vi "AlexeySRS865SweepAC.vi"(0 "VISA resource name":refnum<visa-resource-name>, 1 "Start Ampl":dbl caption="Start, V" format="%^.3e", 2 "Stop Ampl":dbl=1.0 caption="Stop, V" format="%^.5e", 3 "Step Ampl":dbl=0.001 caption="Step, V" format="%^.3e", 4 "Delay (s)":dbl=0.1 format="%.3f", 7 "Start Sweep":bool) -> (5 "Output Ampl":dbl)   [LabVIEW 2025]
doc: "Author: Scott Hannahs <sth@magnet.fsu.edu>\n\nThis software is licensed for use under the “MIT License\"\nCopyright (c) 2025 Scott Hannahs, sth@sth@magnet.sthnet.net\n\nPermission is hereby granted, free of charge, to any person obtaining a copy of this software and associated documentation files (the \"Software\"), to deal in the Software without restriction, including without limitation the rights to use, copy, modify, merge, publish, distribute, sublicense, and/or sell copies of the Software, and to permit persons to whom the Software is furnished to do so, subject to the following conditions: The above copyright notice and this permission notice shall be included in all copies or substantial portions of the Software.\n\nTHE SOFTWARE IS PROVIDED \"AS IS\", WITHOUT WARRANTY OF ANY KIND, EXPRESS OR IMPLIED, INCLUDING BUT NOT LIMITED TO THE WARRANTIES OF MERCHANTABILITY, FITNESS FOR A PARTICULAR PURPOSE AND NONINFRINGEMENT. IN NO EVENT SHALL THE AUTHORS OR COPYRIGHT HOLDERS BE LIABLE FOR ANY CLAIM, DAMAGES OR OTHER LIABILITY, WHETHER IN AN ACTION OF CONTRACT, TORT OR OTHERWISE, ARISING FROM, OUT OF OR IN CONNECTION WITH THE SOFTWARE OR THE USE OR OTHER DEALINGS IN THE SOFTWARE."
panel:
  in  "Pre-steps":dbl=5.0 format="%#_13g"
  in  "SetupBySoft":bool
  out "Calibration\nTime  (sec)":u32 format="%.1f"
  in  "Call Amp INIT":bool
  in  "Stop sweep":bool
  out "Initial Ampl":dbl
  in  "STOP VI":bool
  in  "Output Off":bool
  in  "Setup":bool
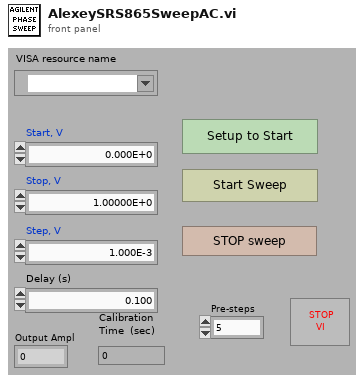
[diagram p1: front panel]
types:
  T1 = enum8{"Enabled", "Disabled", "Disabled and Grayed Out"}
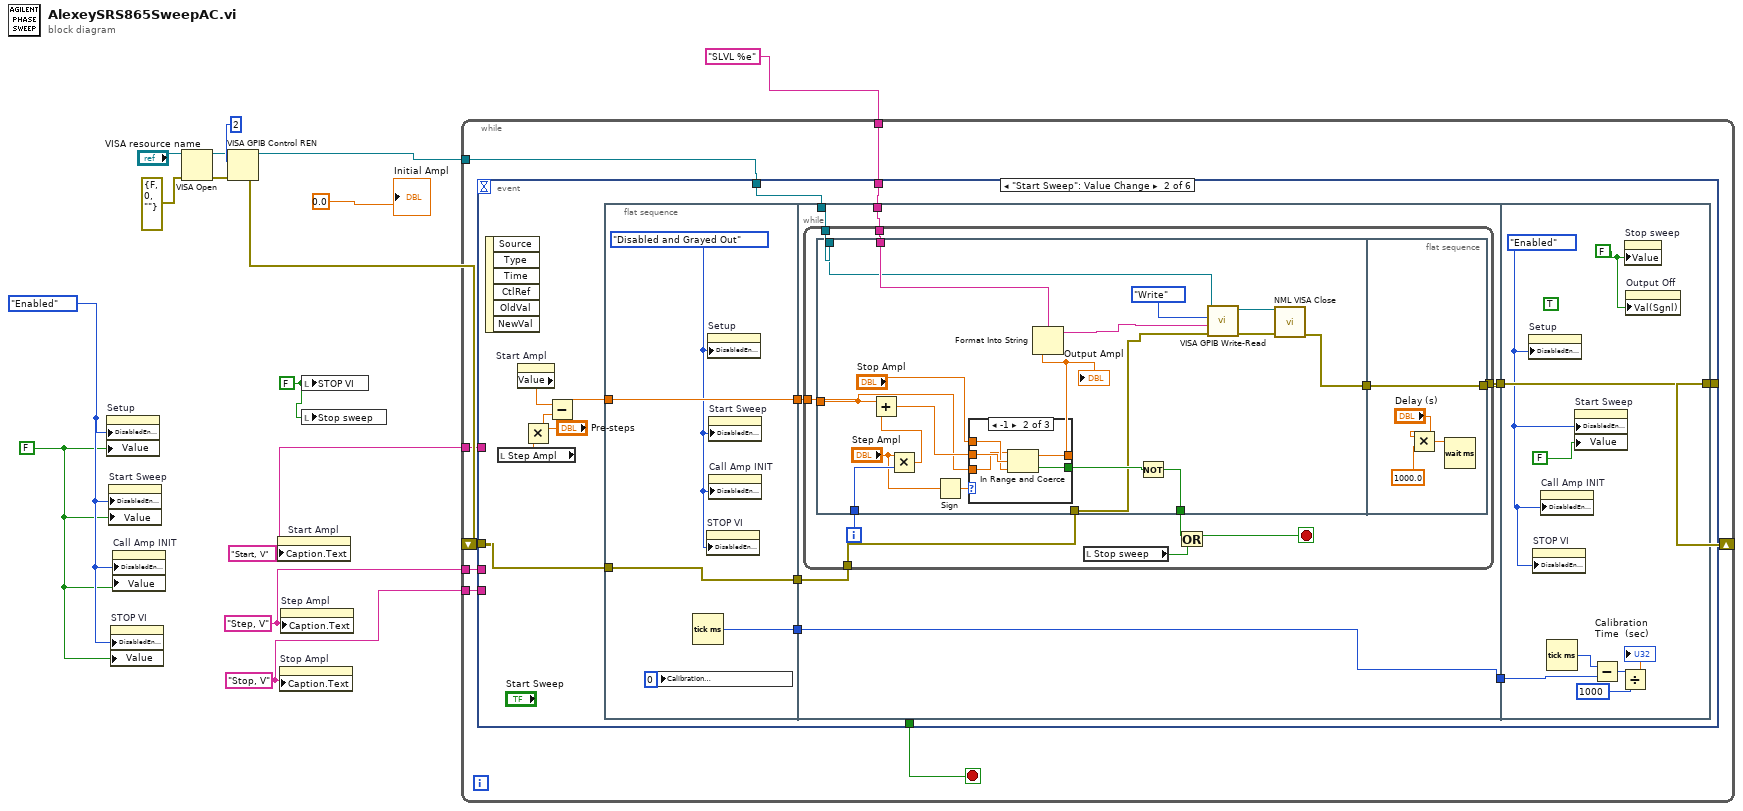
[diagram p0: block diagram]
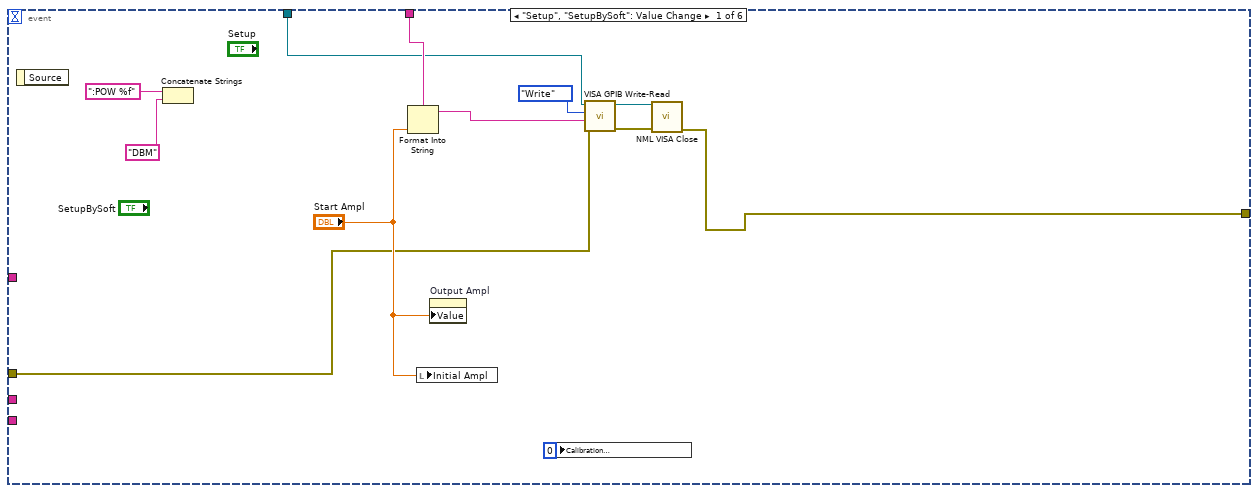
[diagram p2: hidden frame]
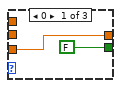
[diagram p3: hidden frame]
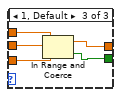
[diagram p4: hidden frame]
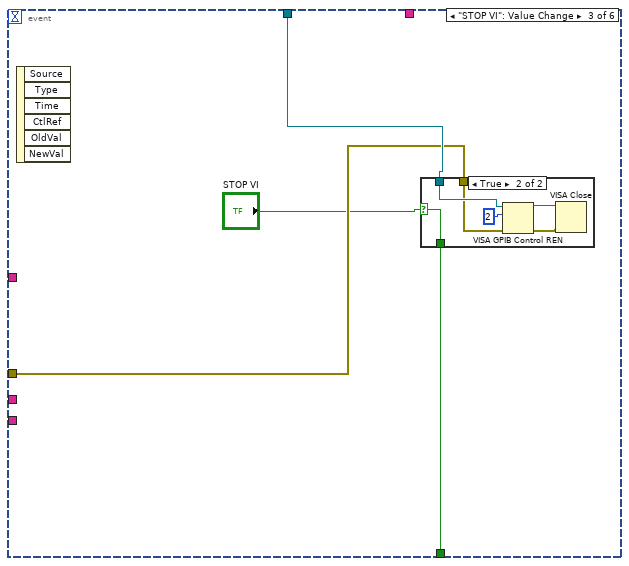
[diagram p5: hidden frame]
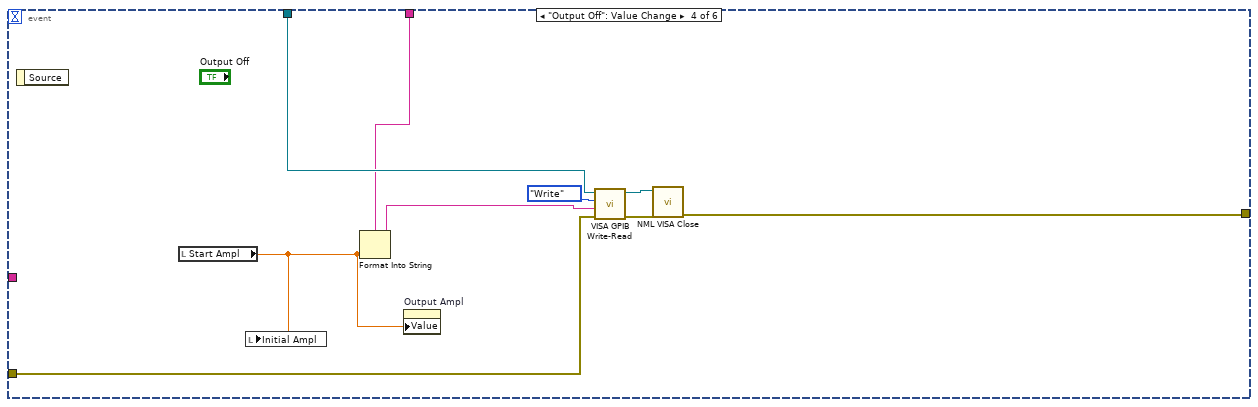
[diagram p7: hidden frame]
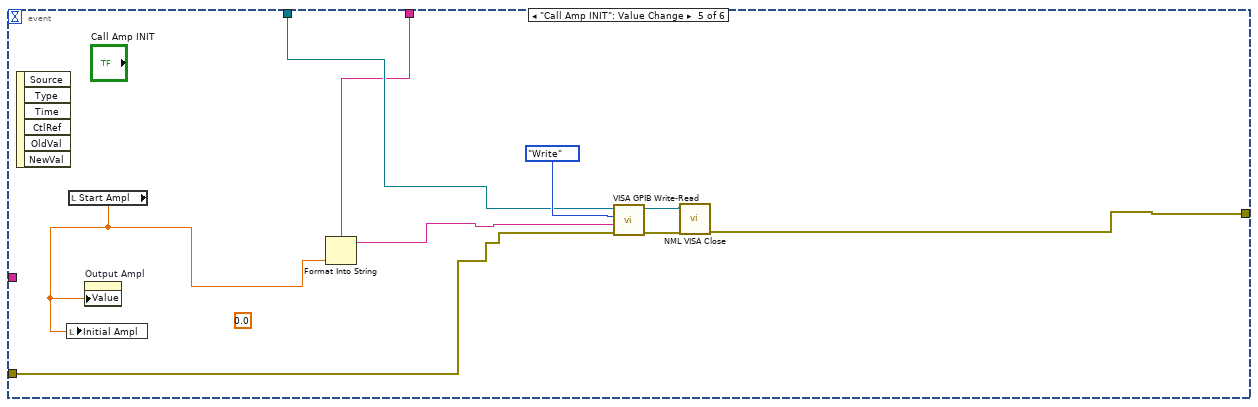
[diagram p8: hidden frame]
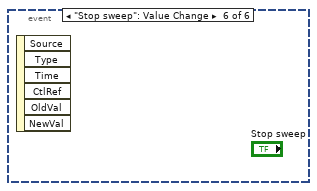
[diagram p9: hidden frame]
diagram:
  w4 = FALSE
  w5 = T1."Enabled" ("Disabled")
  w7 = "Stop, V" ("Label.Text")
  w8 = "Step, V" ("Label.Text")
  w9 = "Start, V" ("Label.Text")
  w6 = FALSE ("NewVal")
  n1 = property on="Setup" class="Bool"("DisabledEnum"=w5, "Value"=w4) -> ()  [unwired: 2 in, 2 out]
  n2 = property on="Start Sweep" class="Bool (strict)"("DisabledEnum"=w5, "Value"=w4) -> ()  [unwired: 2 in, 2 out]
  n3 = property on="STOP VI" class="Bool (strict)"("DisabledEnum"=w5, "Value"=w4) -> ()  [unwired: 2 in, 2 out]
  n4 = property on="Call Amp INIT" class="Bool"("DisabledEnum"=w5, "Value"=w4) -> ()  [unwired: 2 in, 2 out]
  n5 = VISA Open(error in (no error)=errorcluster {"status"=FALSE, "code"=0, "source"=""} ("error out"), VISA resource name="VISA resource name") -> (VISA resource name=w12:refnum<visa-resource-name>, error out=w13:errorcluster)  [unwired: 3 in]
  n6 = VISA GPIB Control REN(8:w13, 10:u16 2 ("mode"), 11:w12) -> (0:w10:errorcluster, 3:w3:refnum<visa-resource-name>)
  n7 = property on="Start Ampl" class="DigNum (strict)"("Caption.Text"=w9) -> ()  [unwired: 2 in, 2 out]
  n8 = property on="Stop Ampl" class="DigNum (strict)"("Caption.Text"=w7) -> ()  [unwired: 2 in, 2 out]
  n9 = property on="Step Ampl" class="DigNum (strict)"("Caption.Text"=w8) -> ()  [unwired: 2 in, 2 out]
  n10 = local write "STOP VI"(w6) -> ()
  n11 = local write "Stop sweep"(w6) -> ()
  n12 = while {
    shift-right: [w21] -> _
    shift-left: w10 -> [w23]
    tunnel: w3 -> [w22]
    tunnel: w9 -> [w19]
    tunnel: w8 -> [w18]
    tunnel: w7 -> [w17]
    tunnel: "SLVL %e" -> [w16]
    stop <- w20 stop-if-true
    n13 = event shown="[1] \"Start Sweep\": Value Change" {
      selector: _ -> [_ _ _ _ _ _]
      dyn-events: _ -> [_ _ _ _ _ _]
      timeout: _ -> [_ _ _ _ _ _]
      tunnel: w22 -> [w27 w49 w117 w133 w139 _]
      tunnel: [w24 w47 _ w125 w134 _] -> w21
      tunnel: w23 -> [w26 w48 w116 w130 w141 _]
      tunnel: [_ _ w114 _ _ _] -> w20
      tunnel: w19 -> [_ _ _ _ _ _]
      tunnel: w18 -> [_ _ _ _ _ _]
      tunnel: w17 -> [_ _ _ _ _ _]
      tunnel: w16 -> [w31 w38 _ w129 w137 _]
      event "Setup", "SetupBySoft": Value Change {
        n14 = event-data() -> ()  [unwired: 1 in, 1 out]
        n15 = Concatenate Strings(":POW %f", "DBM" ("string")) -> ()  [unwired: 1 out]
        n16 = Format Into String(format string=w31, "Start Ampl") -> (resulting string=w25:string)  [unwired: 2 in, 1 out]
        n17 = local write "Initial Ampl"("Start Ampl") -> ()
        n18 = property on="Output Ampl" class="DigNum (strict)"("Value"="Start Ampl") -> ()  [unwired: 2 in, 2 out]
        n19 = local write "Calibration\nTime  (sec)"(u32 0 ("Time Delay (ms)")) -> ()
        n20 = call "VISA GPIB Write-Read.vi"("error in (no error)"=w26, "Command"=w25, "Action"=enum16{"Write", "Read", "Write & Read"}."Write", "VISA resource name"=w27) -> ("error out"=w30:errorcluster, "dup VISA Session"=w29:refnum<visa-resource-name>)  [unwired: 4 in, 2 out]
        n21 = call "NML VISA Close.vi"("Error In"=w30, "VISA resource name"=w29) -> ("Error Out"=w24:errorcluster)  [unwired: 9 in]
      }
      event "Start Sweep": Value Change {
        n22 = event-data() -> ()  [unwired: 1 in, 6 out]
        n23 = local read "Step Ampl"() -> (w39:dbl)
        n24 = property on="Start Ampl" class="DigNum (strict)"() -> ("Value"=w40:dbl)  [unwired: 2 in, 2 out]
        n25 = Multiply(x="Pre-steps", y=w39) -> (x*y=w37:dbl)
        n26 = Subtract(x=w40, y=w37) -> (x-y=w41:dbl)
        n27 = flat-sequence {
          tunnel: w41 -> [w53]
          tunnel: w48 -> [w54]
          tunnel: [w54] -> w45
          tunnel: [w53] -> w44
          tunnel: [w51] -> w43
          tunnel: w49 -> [w60]
          tunnel: [w58] -> w46
          tunnel: w45 -> [w59]
          tunnel: w44 -> [w57]
          tunnel: w43 -> [w56]
          tunnel: [w56] -> w42
          tunnel: w38 -> [w55]
          tunnel: [w113] -> w47
          tunnel: w46 -> [w113]
          tunnel: w42 -> [w110]
          frame #0 {
            w52 = T1."Disabled and Grayed Out" ("Disabled")
            n28 = local write "Calibration\nTime  (sec)"(u32 0 ("Time Delay (ms)")) -> ()
            n29 = Tick Count (ms)() -> (millisecond timer value=w51:u32)
            n30 = property on="STOP VI" class="Bool (strict)"("DisabledEnum"=w52) -> ()  [unwired: 2 in, 2 out]
            n31 = property on="Setup" class="Bool"("DisabledEnum"=w52) -> ()  [unwired: 2 in, 2 out]
            n32 = property on="Start Sweep" class="Bool (strict)"("DisabledEnum"=w52) -> ()  [unwired: 2 in, 2 out]
            n33 = property on="Call Amp INIT" class="Bool"("DisabledEnum"=w52) -> ()  [unwired: 2 in, 2 out]
          }
          frame #1 {
            n34 = while {
              tunnel: w60 -> [w70]
              tunnel: w59 -> [w69]
              tunnel: [w68] -> w58
              tunnel: w57 -> [w67]
              tunnel: w55 -> [w61]
              i -> [w64]
              stop <- w63 stop-if-true
              n35 = flat-sequence {
                tunnel: w70 -> [w72]
                tunnel: w69 -> [w74]
                tunnel: w67 -> [w80]
                tunnel: [w88] -> w66
                tunnel: [w75] -> w65
                tunnel: w64 -> [w87]
                tunnel: w61 -> [w78]
                tunnel: [w104] -> w68
                tunnel: w65 -> [w104]
                frame #0 {
                  n36 = Multiply(x="Step Ampl", y=w87) -> (x*y=w86:dbl)
                  n37 = Add(x=w80, y=w86) -> (x+y=w82:dbl)
                  n38 = Sign(1:"Step Ampl") -> (0:w85:dbl)
                  n39 = case shown="-1" w85 {
                    tunnel: [FALSE w95 w96] -> w84
                    tunnel: [w90 w94 w97] -> w83
                    tunnel: w82 -> [_ w93 w100]
                    tunnel: "Stop Ampl" -> [_ w92 w99]
                    tunnel: w80 -> [w90 w91 w98]
                    frame 0 {
                    }
                    frame -1 {
                      n40 = In Range and Coerce(upper limit=w91, x=w93, lower limit=w92) -> (coerced(x)=w94:dbl, In Range?=w95:bool)
                    }
                    frame 1, Default {
                      n41 = In Range and Coerce(upper limit=w99, x=w100, lower limit=w98) -> (coerced(x)=w97:dbl, In Range?=w96:bool)
                    }
                  }
                  "Output Ampl" <- w83
                  n42 = Format Into String(format string=w78, w83) -> (resulting string=w73:string)  [unwired: 2 in, 1 out]
                  n43 = Not(x=w84) -> (.not. x?=w88:bool)
                  n44 = call "VISA GPIB Write-Read.vi"("error in (no error)"=w74, "Command"=w73, "Action"=enum16{"Write", "Read", "Write & Read"}."Write", "VISA resource name"=w72) -> ("error out"=w77:errorcluster, "dup VISA Session"=w76:refnum<visa-resource-name>)  [unwired: 4 in, 2 out]
                  n45 = call "NML VISA Close.vi"("Error In"=w77, "VISA resource name"=w76) -> ("Error Out"=w75:errorcluster)  [unwired: 9 in]
                }
                frame #1 {
                  n46 = Multiply(x="Delay (s)", y=1000.0) -> (x*y=w102:dbl)
                  n47 = Wait (ms)(milliseconds to wait=w102) -> ()  [unwired: 1 out]
                }
              }
              n48 = local read "Stop sweep"() -> (w62:bool)
              n49 = Or(x=w66, y=w62) -> (x .or. y?=w63:bool)
            }
          }
          frame #2 {
            w105 = FALSE ("Stop sweep")
            w112 = T1."Enabled" ("Disabled")
            (unwired) TRUE ("DEG\n\nRad")
            n50 = property on="Setup" class="Bool"("DisabledEnum"=w112) -> ()  [unwired: 2 in, 2 out]
            n51 = property on="STOP VI" class="Bool (strict)"("DisabledEnum"=w112) -> ()  [unwired: 2 in, 2 out]
            n52 = property on="Call Amp INIT" class="Bool"("DisabledEnum"=w112) -> ()  [unwired: 2 in, 2 out]
            n53 = Tick Count (ms)() -> (millisecond timer value=w111:u32)
            n54 = property on="Start Sweep" class="Bool (strict)"("DisabledEnum"=w112, "Value"=FALSE) -> ()  [unwired: 2 in, 2 out]
            n55 = Subtract(x=w111, y=w110) -> (x-y=w108:u32)
            n56 = Divide(x=w108, y=u32 1000) -> (x/y=→"Calibration\nTime  (sec)":dbl)
            n57 = property on="Stop sweep" class="Bool (strict)"("Value"=w105) -> ()  [unwired: 2 in, 2 out]
            n58 = property on="Output Off" class="Bool (strict)"("Val(Sgnl)"=w105) -> ()  [unwired: 2 in, 2 out]
          }
        }
      }
      event "STOP VI": Value Change {
        n59 = event-data() -> ()  [unwired: 1 in, 6 out]
        n60 = case shown="True" "STOP VI" {
          selector: "STOP VI" -> [w118 w124]
          tunnel: [w118 w124] -> w114
          tunnel: w117 -> [_ w121]
          tunnel: w116 -> [_ w120]
          frame False {
          }
          frame True {
            n61 = VISA GPIB Control REN(8:w120, 10:u16 2 ("mode"), 11:w121) -> (0:w119:errorcluster, 3:w122:refnum<visa-resource-name>)
            n62 = VISA Close(VISA resource name=w122, error in (no error)=w119) -> ()  [unwired: 1 out]
          }
        }
      }
      event "Output Off": Value Change {
        n63 = event-data() -> ()  [unwired: 1 in, 1 out]
        n64 = local read "Start Ampl"() -> (w128:dbl)
        n65 = local write "Initial Ampl"(w128) -> ()
        n66 = Format Into String(format string=w129, w128) -> (resulting string=w131:string)  [unwired: 2 in, 1 out]
        n67 = property on="Output Ampl" class="DigNum (strict)"("Value"=w128) -> ()  [unwired: 2 in, 2 out]
        n68 = call "VISA GPIB Write-Read.vi"("error in (no error)"=w130, "Command"=w131, "Action"=enum16{"Write", "Read", "Write & Read"}."Write", "VISA resource name"=w133) -> ("error out"=w126:errorcluster, "dup VISA Session"=w127:refnum<visa-resource-name>)  [unwired: 4 in, 2 out]
        n69 = call "NML VISA Close.vi"("Error In"=w126, "VISA resource name"=w127) -> ("Error Out"=w125:errorcluster)  [unwired: 9 in]
      }
      event "Call Amp INIT": Value Change {
        (unwired) 0.0 ("Output Phase")
        n70 = event-data() -> ()  [unwired: 1 in, 6 out]
        n71 = local read "Start Ampl"() -> (w138:dbl)
        n72 = local write "Initial Ampl"(w138) -> ()
        n73 = property on="Output Ampl" class="DigNum (strict)"("Value"=w138) -> ()  [unwired: 2 in, 2 out]
        n74 = Format Into String(format string=w137, w138) -> (resulting string=w140:string)  [unwired: 2 in, 1 out]
        n75 = call "VISA GPIB Write-Read.vi"("error in (no error)"=w141, "Command"=w140, "Action"=enum16{"Write", "Read", "Write & Read"}."Write", "VISA resource name"=w139) -> ("error out"=w135:errorcluster, "dup VISA Session"=w136:refnum<visa-resource-name>)  [unwired: 4 in, 2 out]
        n76 = call "NML VISA Close.vi"("Error In"=w135, "VISA resource name"=w136) -> ("Error Out"=w134:errorcluster)  [unwired: 9 in]
      }
      event "Stop sweep": Value Change {
        n77 = event-data() -> ()  [unwired: 1 in, 6 out]
      }
    }
  }
  "Initial Ampl" <- 0.0 ("Initial Ampl")
